vi "CD Read Engine_Parse Message.vi"(8 "Error (in)":errorcluster, 9 "Inline Status Channels Refs":T1[](array[typedef]) format="%.0x", 10 "Record []":T11[](array[typedef]) {"type" format="%04x"; "activity" format="%04x"; "error" format="%04x"; "cwd1" format="%04x"; "cwd2" format="%04x"; "swd1" format="%04x"; "swd2" format="%04x"; "data" format="%04x"}, 11 "RT Inline Data_Data Description_Channels":T2[](array[typedef]) {"Frame Drescriptors"."RT"."Status Channel Ref" format="%.0x"; "Frame Drescriptors"."RT"."Words Block Data Refs"."Data Reference" format="%.0x"; "Frame Drescriptors"."RT"."Timestamp Channel Data Reference" format="%.0x"; "Frame Drescriptors"."BC"."Status Channel Refs" format="%.0x"; "Frame Drescriptors"."BC"."Words Block Data Refs"."Data Reference" format="%.0x"; "Frame Drescriptors"."BC"."Timestamp Channel Data Reference" format="%.0x"}) -> (0 "Error (out)":errorcluster)   [LabVIEW 2017, in "Ballard MIL-1553 Engine.lvlib"]
uses:
  Ballard MIL-1553 Engine.lvlib
  <instrlib>/BTICardLib/Public/Controls/1553 Record.ctl
  Controls/RT Inline Data_Data Description_Channel.ctl
  Controls/RT Inline Frame Descriptor.ctl
  Controls/RT Inline Frame Descriptor_BC.ctl
  <vilib>/NI Veristand/Custom Device API/Data Reference.ctl
  <vilib>/NI Veristand/Custom Device API/Block Data Reference.ctl
  <vilib>/NI Veristand/Custom Device API/Custom Device Item Ref.ctl
  Controls/RT Inline Frame Descriptor_RT.ctl
  Shared/Controls and Global/RT CWD2.ctl
  Shared/Controls and Global/RT CWD1.ctl
  Shared/Controls and Global/RT messageType.ctl
  <vilib>/NI VeriStand/Custom Device Tools/Custom Device Utility Library/Custom Device Utility Library.lvlib
  <vilib>/NI VeriStand/Custom Device API/Custom Device API.lvlib
  <instrlib>/BTICardLib/BTICardLV.lvlib
  Shared/Ballard 1553 Shared.lvlib
panel:
  out "Physical Channel":u16
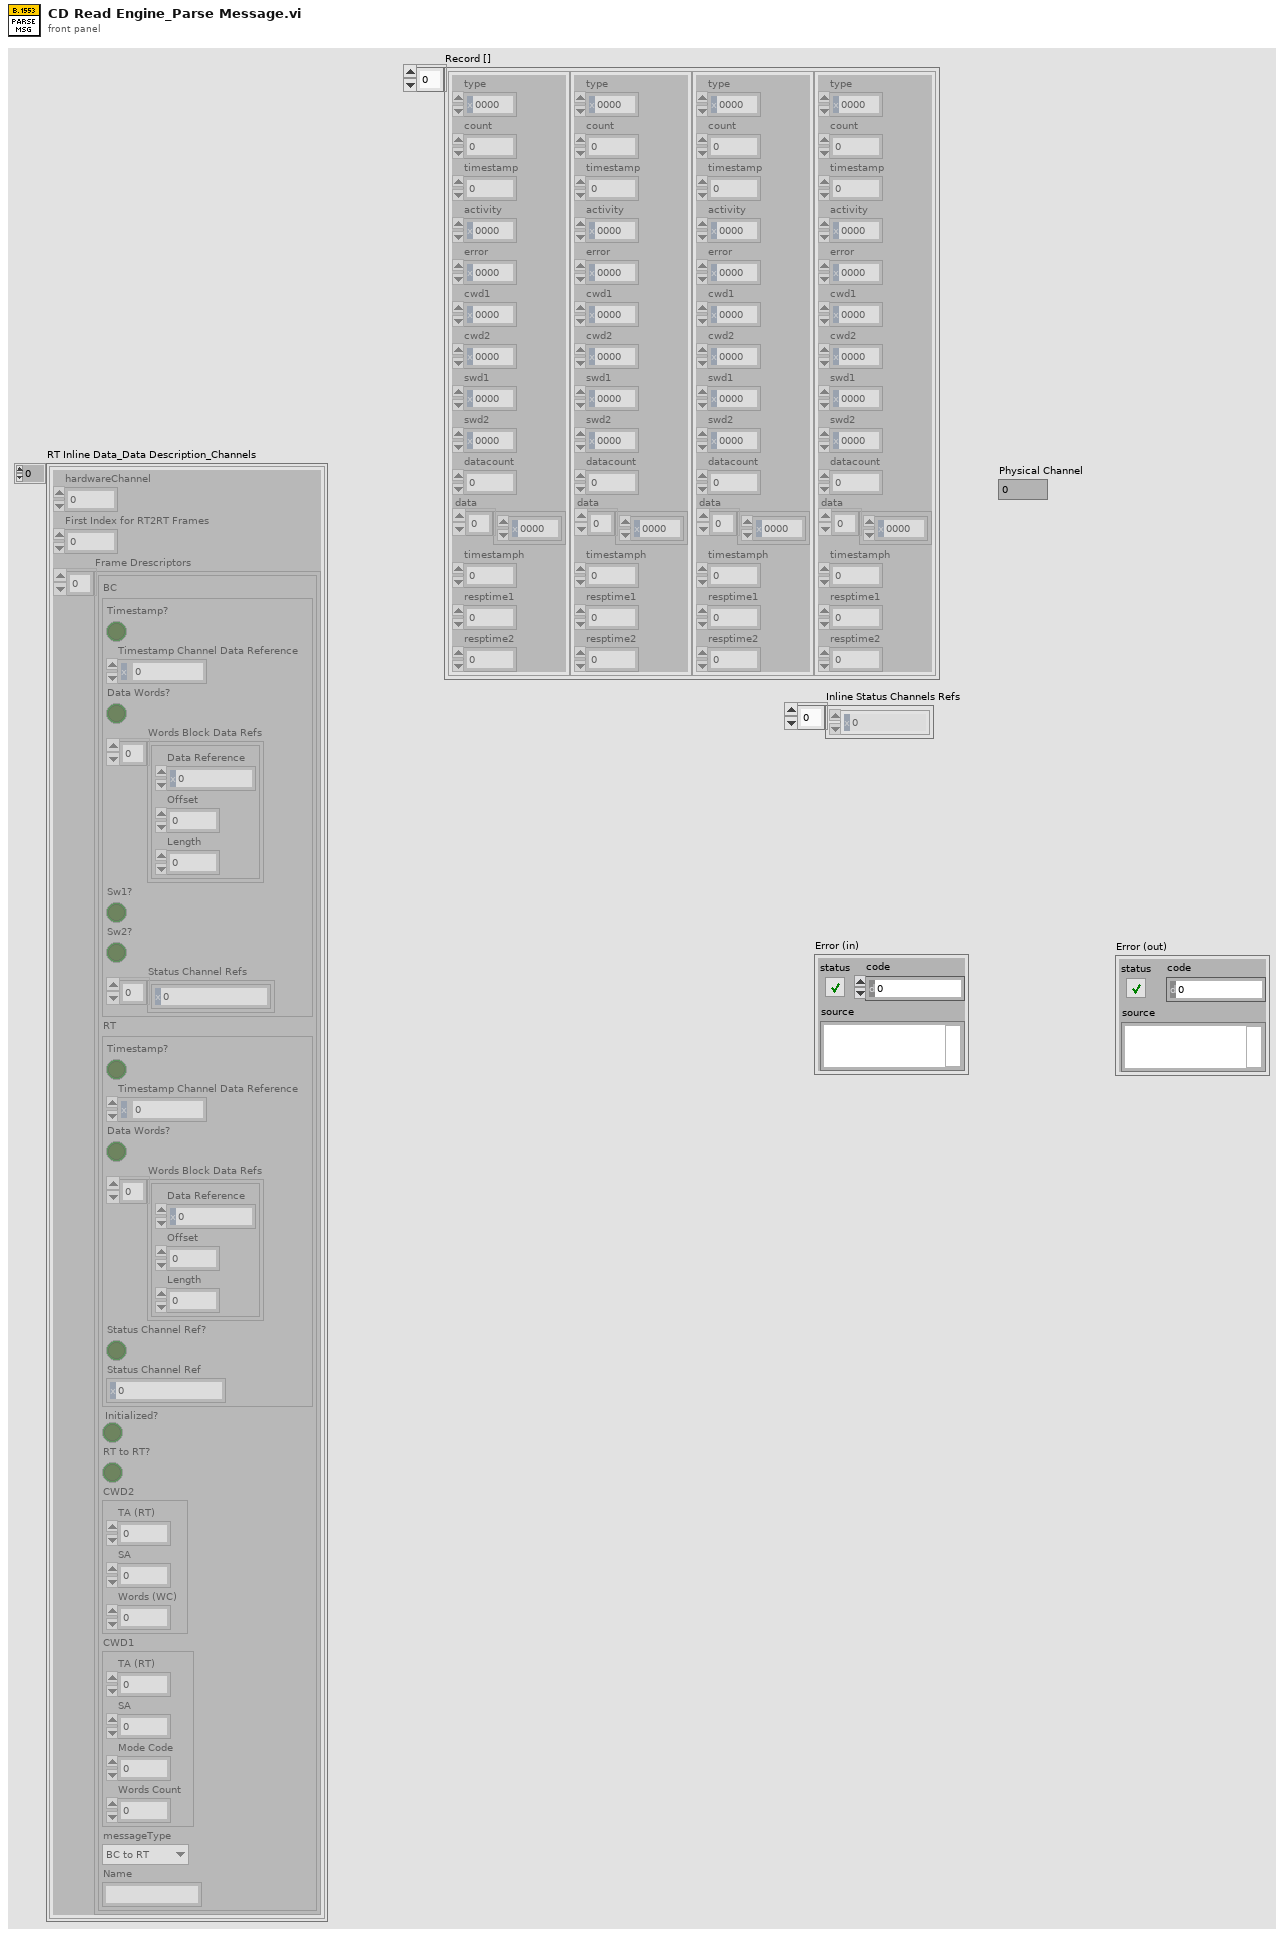
[diagram p1: front panel]
types:
  T1 = typedef "Custom Device API.lvlib/Data Reference.ctl" = i32
  T2 = typedef "Ballard MIL-1553 Engine.lvlib/RT Inline Data_Data Description_Channel.ctl" = cluster{"hardwareChannel":u16, "First Index for RT2RT Frames":i32, "Frame Drescriptors":T3[]}
  T3 = typedef "Ballard MIL-1553 Engine.lvlib/RT Inline Frame Descriptor.ctl" = cluster{"BC":T4, "RT":T7, "Initialized?":bool, "RT to RT?":bool, "CWD2":T8, "CWD1":T9, "messageType":T10, "Name":string}
  T4 = typedef "Ballard MIL-1553 Engine.lvlib/RT Inline Frame Descriptor_BC.ctl" = cluster{"Timestamp?":bool, "Timestamp Channel Data Reference":T1, "Data Words?":bool, "Words Block Data Refs":T5[], "Sw1?":bool, "Sw2?":bool, "Status Channel Refs":T6[]}
  T5 = typedef "Custom Device API.lvlib/Block Data Reference.ctl" = cluster{"Data Reference":T1, "Offset":u64, "Length":u64}
  T6 = typedef "Custom Device API.lvlib/Custom Device Item Ref.ctl" = u64
  T7 = typedef "Ballard MIL-1553 Engine.lvlib/RT Inline Frame Descriptor_RT.ctl" = cluster{"Timestamp?":bool, "Timestamp Channel Data Reference":T1, "Data Words?":bool, "Words Block Data Refs":T5[], "Status Channel Ref?":bool, "Status Channel Ref":T6}
  T8 = typedef "Ballard 1553 Shared.lvlib/RT CWD2.ctl" = cluster{"TA (RT)":i8, "SA":i8, "Words (WC)":i8}
  T9 = typedef "Ballard 1553 Shared.lvlib/RT CWD1.ctl" = cluster{"TA (RT)":i8, "SA":i8, "Mode Code":i8, "Words Count":i8}
  T10 = typedef "Ballard 1553 Shared.lvlib/RT messageType.ctl" = enum16{"BC to RT", "RT to BC", "RT to RT", "MC (Rx)", "MC (Tx)"}
  T11 = typedef "BTICardLV.lvlib/1553 Record.ctl" = cluster{"type":u16, "count":u16, "timestamp":u32, "activity":u16, "error":u16, "cwd1":u16, "cwd2":u16, "swd1":u16, "swd2":u16, "datacount":u16, "data":u16[], "timestamph":u32, "resptime1":u16, "resptime2":u16}
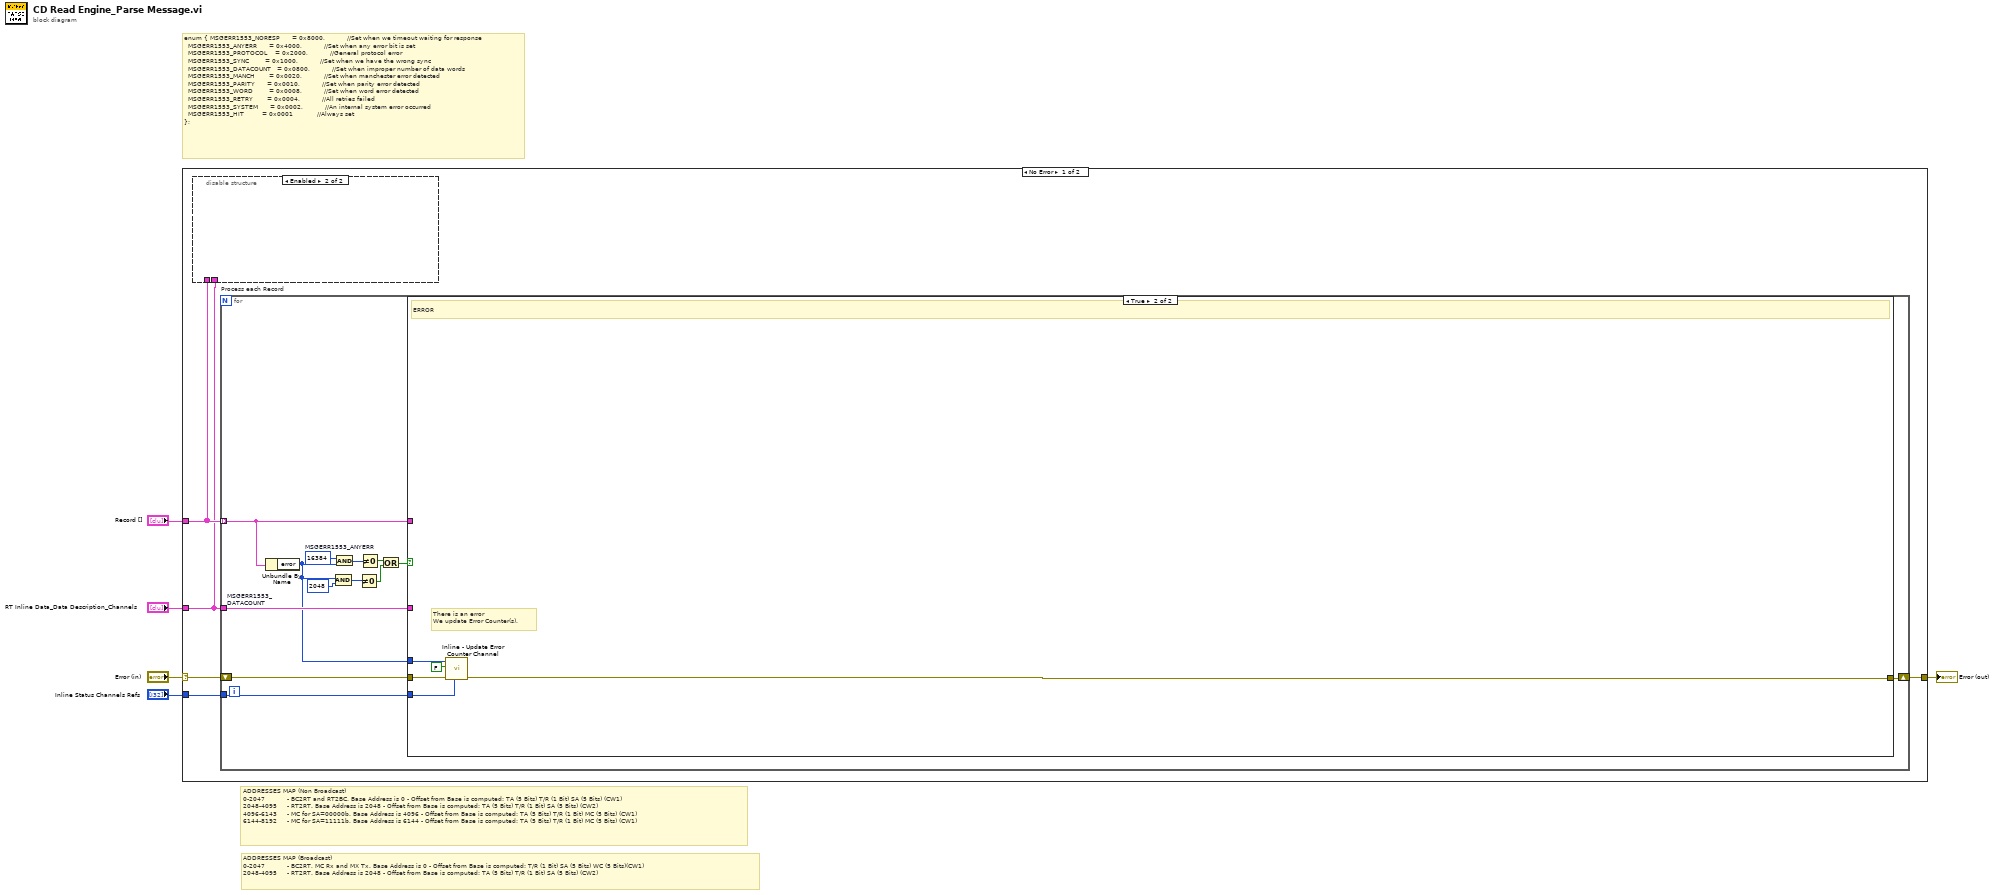
[diagram p0: block diagram]
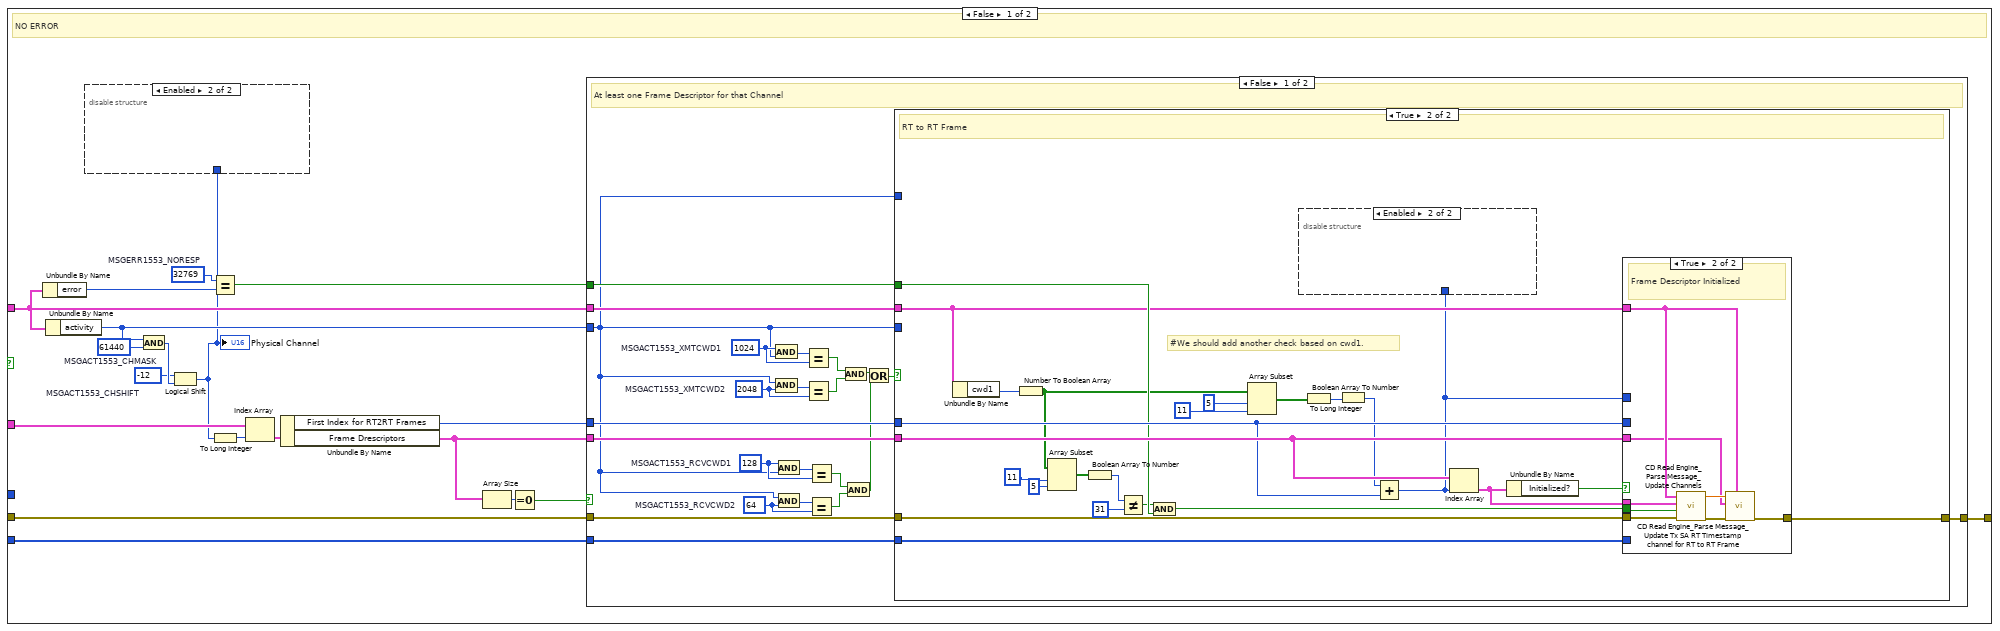
[diagram p2: hidden frame]
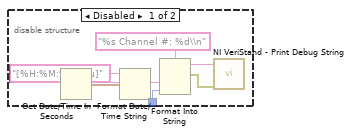
[diagram p3: hidden frame]
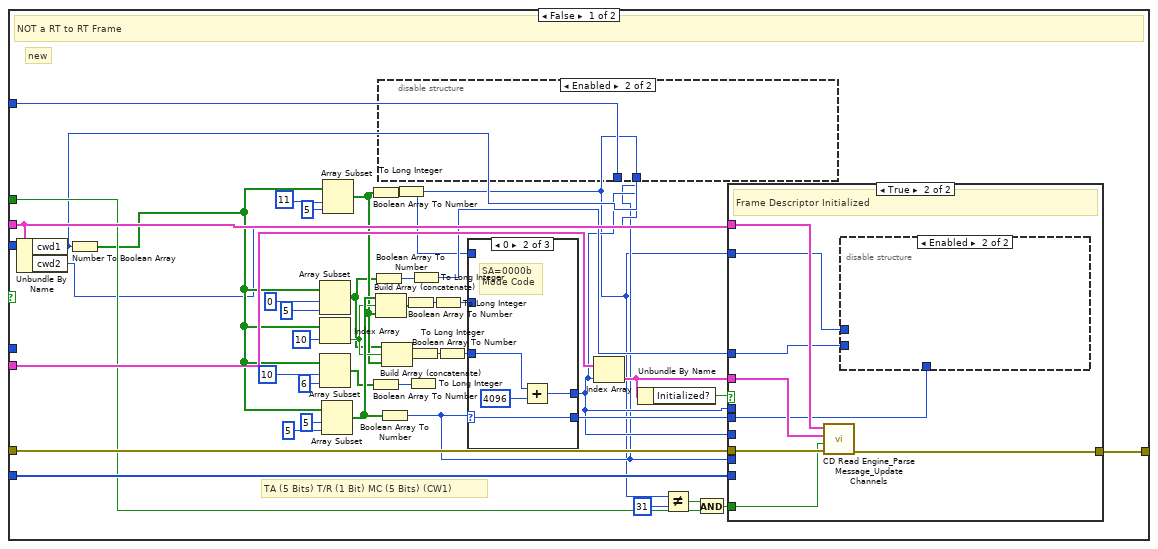
[diagram p4: hidden frame]
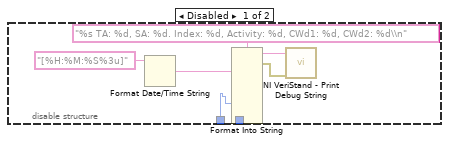
[diagram p5: hidden frame]
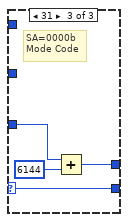
[diagram p7: hidden frame]
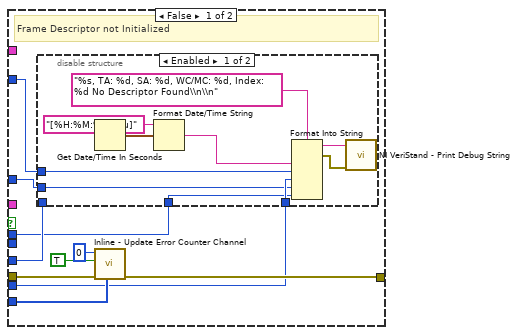
[diagram p8: hidden frame]
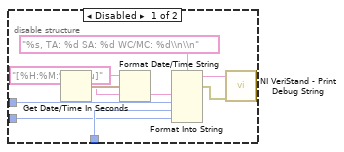
[diagram p10: hidden frame]
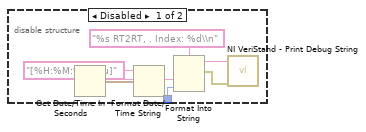
[diagram p11: hidden frame]
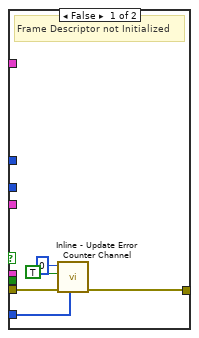
[diagram p12: hidden frame]
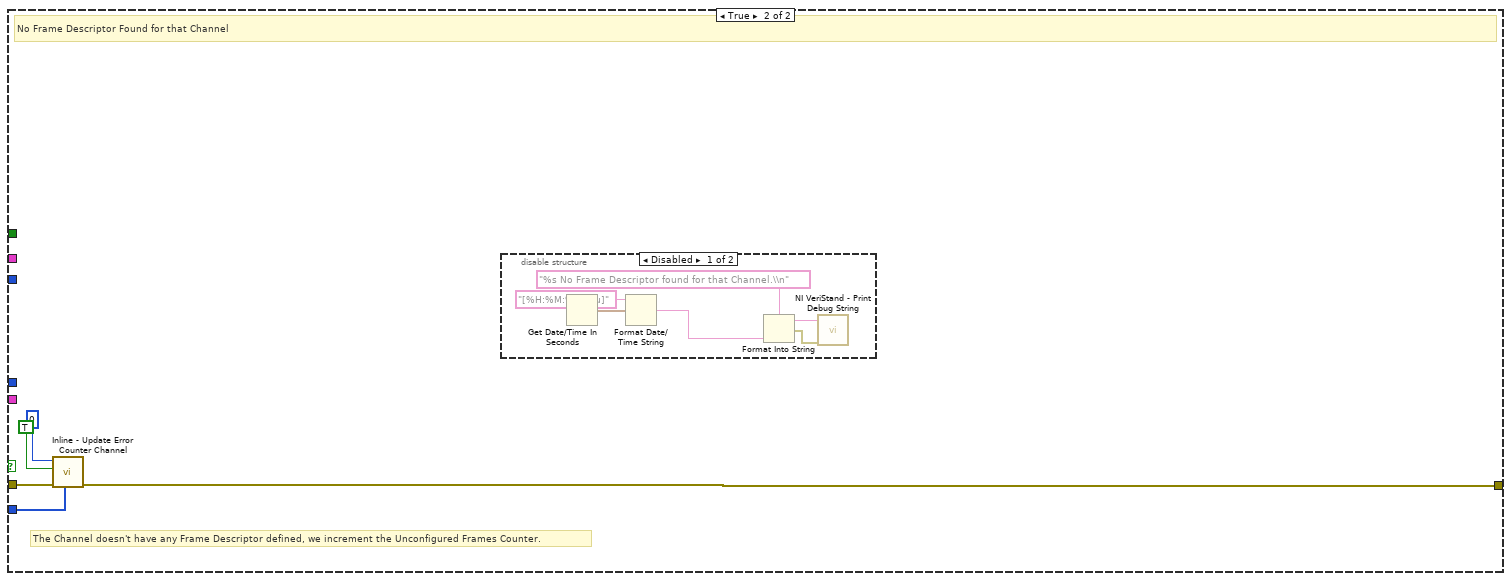
[diagram p13: hidden frame]
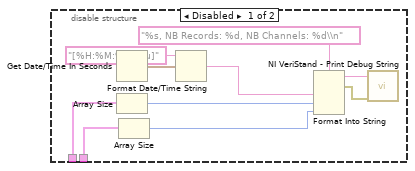
[diagram p15: hidden frame]
diagram:
  # "ADDRESSES MAP (Broadcast) \n0-2047           - BC2RT, MC Rx and MX Tx. Base Address is 0 - Offset from Base is computed: T/R (1 Bit) SA (5 Bits) WC (5 Bits)(CW1)\n2048-4095     - RT2RT. Base Address is 2048 - Offset from Base is computed: TA (5 Bits) T/R (1 Bit) SA (5 Bits) (CW2)"
  # "ADDRESSES MAP (Non Broadcast) \n0-2047           - BC2RT and RT2BC. Base Address is 0 - Offset from Base is computed: TA (5 Bits) T/R (1 Bit) SA (5 Bits) (CW1)\n2048-4095     - RT2RT. Base Address is 2048 - Offset from Base is computed: TA (5 Bits) T/R (1 Bit) SA (5 Bits) (CW2)\n4096-6143     - MC for SA=00000b. Base Address is 4096 - Offset from Base is computed: TA (5 Bits) T/R (1 Bit) MC (5 Bits) (CW1)\n6144-8192     - MC for SA=11111b. Base Address is 6144 - Offset from Base is computed: TA (5 Bits) T/R (1 Bit) MC (5 Bits) (CW1)"
  # "enum {\tMSGERR1553_NORESP      = 0x8000,           //Set when we timeout waiting for response\n\t\tMSGERR1553_ANYERR      = 0x4000,           //Set when any error bit is set\n\t\tMSGERR1553_PROTOCOL    = 0x2000,           //General protocol error\n\t\tMSGERR1553_SYNC        = 0x1000,           //Set when we have the wrong sync\n\t\tMSGERR1553_DATACOUNT   = 0x0800,           //Set when improper number of data words\n\t\tMSGERR1553_MANCH       = 0x0020,           //Set when manchester error detected\n\t\tMSGERR1553_PARITY      = 0x0010,           //Set when parity error detected\n\t\tMSGERR1553_WORD        = 0x0008,           //Set when word error detected\n\t\tMSGERR1553_RETRY       = 0x0004,           //All retries failed\n\t\tMSGERR1553_SYSTEM      = 0x0002,           //An internal system error occurred\n\t\tMSGERR1553_HIT         = 0x0001            //Always set\n};"
  n1 = case shown="No Error" "Error (in)" {
    selector: "Error (in)" -> [w9 w244]
    tunnel: "Record []" -> [w8 _]
    tunnel: [w10 w244] -> w4
    tunnel: "RT Inline Data_Data Description_Channels" -> [w6 _]
    tunnel: "Inline Status Channels Refs" -> [w7 _]
    frame No Error {
      n2 = disable-structure shown="Enabled" {
        disable-tunnel: w8 -> [w243 _]
        disable-tunnel: w6 -> [w235 _]
        frame Disabled {
          n3 = Get Date/Time In Seconds() -> (seconds since 1Jan1904=w242:timestamp)
          n4 = Array Size(array=w243) -> (size(s)=w240:i32)
          n5 = Array Size(array=w235) -> (size(s)=w234:i32)
          n6 = Format Date/Time String(time format string (%c)="[%H:%M:%S%3u]", seconds (now)=w242) -> (date/time string=w241:string)  [unwired: 1 in]
          n7 = Format Into String(format string="%s, NB Records: %d, NB Channels: %d\\n", w241, w240, w234) -> (resulting string=w236:string, error out=w237:errorcluster)  [unwired: 2 in]
          n8 = call <vilib>:"NI VeriStand - Print Debug String.vi"("error in (no error)"=w237, "Message"=w236) -> ()  [unwired: 9 in, 1 out]
        }
        frame Enabled {
        }
      }
      n9 = for "Process each Record" {
        tunnel: w8 -> [w23] mode=indexing
        shift-right: [w22] -> w10
        shift-left: w9 -> [w21]
        tunnel: w7 -> [w20]
        tunnel: w6 -> [w19]
        w11 = u16 2048  # MSGERR1553_DATACOUNT
        w18 = u16 16384  # MSGERR1553_ANYERR
        n10 = Unbundle By Name(w23) -> ("error"=w14:u16)
        n11 = And(x=w14, y=w11) -> (x .and. y?=w13:u16)
        n12 = And(x=w18, y=w14) -> (x .and. y?=w17:u16)
        n13 = Not Equal To 0?(x=w13) -> (x != 0?=w12:bool)
        n14 = Not Equal To 0?(x=w17) -> (x != 0?=w16:bool)
        n15 = Or(x=w16, y=w12) -> (x .or. y?=w15:bool)
        n16 = case "Channel Found?" shown="True" w15 {
          tunnel: w21 -> [w41 w232]
          tunnel: [w42 w230] -> w22
          tunnel: w23 -> [w29 _]
          tunnel: w20 -> [w32 w231]
          tunnel: w19 -> [w39 _]
          tunnel: w14 -> [_ w233]
          frame False {
            w27 = u16 32769  # MSGERR1553_NORESP
            w30 = i16 -12  # MSGACT1553_CHSHIFT
            w40 = u16 61440  # MSGACT1553_CHMASK
            # "NO ERROR"
            n17 = Unbundle By Name(w29) -> ("error"=w28:u16)
            n18 = Unbundle By Name(w29) -> ("activity"=w34:u16)
            n19 = And(x=w34, y=w40) -> (x .and. y?=w31:u16)
            n20 = Logical Shift(y=w30, x=w31) -> (x << y=w25:u16)
            "Physical Channel" <- w25
            n21 = disable-structure shown="Enabled" {
              disable-tunnel: w25 -> [w43 _]
              frame Disabled {
                n22 = Get Date/Time In Seconds() -> (seconds since 1Jan1904=w49:timestamp)
                n23 = Format Date/Time String(time format string (%c)="[%H:%M:%S%3u]", seconds (now)=w49) -> (date/time string=w48:string)  [unwired: 1 in]
                n24 = Format Into String(format string="%s Channel #: %d\\n", w48, w43) -> (resulting string=w44:string, error out=w45:errorcluster)  [unwired: 2 in]
                n25 = call <vilib>:"NI VeriStand - Print Debug String.vi"("error in (no error)"=w45, "Message"=w44) -> ()  [unwired: 9 in, 1 out]
              }
              frame Enabled {
              }
            }
            n26 = Equal?(x=w27, y=w28) -> (x = y?=w26:bool)
            n27 = To Long Integer(number=w25) -> (32bit integer=w38:i32)
            n28 = Index Array(array=w39, index=w38) -> (element=w36:T2)
            n29 = Unbundle By Name(w36) -> ("First Index for RT2RT Frames"=w33:i32, "Frame Drescriptors"=w35:T3[])
            n30 = Array Size(array=w35) -> (size(s)=w37:i32)
            n31 = Equal To 0?(x=w37) -> (x = 0?=w24:bool)
            n32 = case shown="False" w24 {
              tunnel: [w72 w218] -> w42
              tunnel: w29 -> [w71 _]
              tunnel: w41 -> [w70 w221]
              tunnel: w35 -> [w63 _]
              tunnel: w34 -> [w50 _]
              tunnel: w33 -> [w64 _]
              tunnel: w32 -> [w62 w220]
              tunnel: w26 -> [w60 _]
              frame False {
                w59 = u16 128  # MSGACT1553_RCVCWD1
                w58 = u16 64  # MSGACT1553_RCVCWD2
                w61 = u16 1024  # MSGACT1553_XMTCWD1
                w65 = u16 2048  # MSGACT1553_XMTCWD2
                # "At least one Frame Descriptor for that Channel"
                n33 = And(x=w61, y=w50) -> (x .and. y?=w68:u16)
                n34 = And(x=w50, y=w65) -> (x .and. y?=w66:u16)
                n35 = And(x=w59, y=w50) -> (x .and. y?=w55:u16)
                n36 = And(x=w50, y=w58) -> (x .and. y?=w57:u16)
                n37 = Equal?(x=w68, y=w61) -> (x = y?=w69:bool)
                n38 = Equal?(x=w66, y=w65) -> (x = y?=w67:bool)
                n39 = Equal?(x=w55, y=w59) -> (x = y?=w54:bool)
                n40 = Equal?(x=w57, y=w58) -> (x = y?=w56:bool)
                n41 = And(x=w69, y=w67) -> (x .and. y?=w52:bool)
                n42 = And(x=w54, y=w56) -> (x .and. y?=w51:bool)
                n43 = Or(x=w52, y=w51) -> (x .or. y?=w53:bool)
                n44 = case shown="True" w53 {
                  tunnel: w71 -> [w113 w191]
                  tunnel: w70 -> [w114 w196]
                  tunnel: [w115 w197] -> w72
                  tunnel: w64 -> [_ w193]
                  tunnel: w63 -> [w112 w195]
                  tunnel: w62 -> [w111 w194]
                  tunnel: w60 -> [w110 w192]
                  tunnel: w50 -> [_ _]
                  tunnel: w50 -> [w109 _]
                  frame False {
                    # "TA (5 Bits) T/R (1 Bit) MC (5 Bits) (CW1)"
                    # "new"
                    # "NOT a RT to RT Frame"
                    n45 = Unbundle By Name(w113) -> ("cwd1"=w107:u16, "cwd2"=w106:u16)
                    n46 = Number To Boolean Array(number=w107) -> (Boolean array=w108:bool[])
                    n47 = Array Subset(array=w108, index=0, length=5) -> (w81:bool[])
                    n48 = Index Array(array=w108, index=10) -> (element=w84:bool)
                    n49 = Array Subset(array=w108, index=10, length=6) -> (w79:bool[])
                    n50 = Array Subset(array=w108, index=5, length=5) -> (w85:bool[])
                    n51 = Array Subset(array=w108, index=11, length=5) -> (w83:bool[])
                    n52 = Boolean Array To Number(Boolean array=w83) -> (number=w90:u32)
                    n53 = Boolean Array To Number(Boolean array=w79) -> (number=w80:u32)
                    n54 = Boolean Array To Number(Boolean array=w81) -> (number=w94:u32)
                    n55 = Build Array (concatenate)(w85, w84, w83) -> (w99:bool[])
                    n56 = Boolean Array To Number(Boolean array=w85) -> (number=w77:u16)
                    n57 = Build Array (concatenate)(w81, w84, w83) -> (w82:bool[])
                    n58 = To Long Integer(number=w90) -> (32bit integer=w75:i32)
                    n59 = Boolean Array To Number(Boolean array=w99) -> (number=w96:u16)
                    n60 = To Long Integer(number=w80) -> ()  [unwired: 1 out]
                    n61 = Boolean Array To Number(Boolean array=w82) -> (number=w87:u16)
                    n62 = To Long Integer(number=w94) -> (32bit integer=w93:i32)
                    n63 = To Long Integer(number=w96) -> (32bit integer=w89:i32)
                    n64 = To Long Integer(number=w87) -> (32bit integer=w86:i32)
                    n65 = case shown="0" w77 {
                      selector: w77 -> [w128 w130 w134]
                      tunnel: w75 -> [_ _ _]
                      tunnel: [w127 w132 w136] -> w78
                      tunnel: w89 -> [w127 _ _]
                      tunnel: [w128 w130 w134] -> w95
                      tunnel: w86 -> [_ w129 w133]
                      frame 1, Default {
                      }
                      frame 0 {
                        # "SA=0000b\nMode Code"
                        n66 = Add(x=w129, y=4096) -> (x+y=w132:i32)
                      }
                      frame 31 {
                        # "SA=0000b\nMode Code"
                        n67 = Add(x=w133, y=6144) -> (x+y=w136:i32)
                      }
                    }
                    n68 = disable-structure shown="Enabled" {
                      disable-tunnel: w75 -> [w122 _]
                      disable-tunnel: w78 -> [w121 _]
                      disable-tunnel: w77 -> [w119 _]
                      disable-tunnel: w109 -> [w118 _]
                      disable-tunnel: w107 -> [w117 _]
                      disable-tunnel: w106 -> [w116 _]
                      frame Disabled {
                        n69 = Format Date/Time String(time format string (%c)="[%H:%M:%S%3u]") -> (date/time string=w126:string)  [unwired: 2 in]
                        n70 = Format Into String(format string="%s TA: %d, SA: %d. Index: %d, Activity: %d, CWd1: %d, CWd2: %d\\n", w126, w122, w119, w121, w118, w117, w116) -> (resulting string=w123:string, error out=w124:errorcluster)  [unwired: 2 in]
                        n71 = call <vilib>:"NI VeriStand - Print Debug String.vi"("error in (no error)"=w124, "Message"=w123) -> ()  [unwired: 9 in, 1 out]
                      }
                      frame Enabled {
                      }
                    }
                    n72 = Index Array(array=w112, index=w78) -> (element=w105:T3)
                    n73 = Unbundle By Name(w105) -> ("Initialized?"=w104:bool)
                    n74 = Not Equal?(x=w75, y=31) -> (x != y?=w76:bool)
                    n75 = And(x=w76, y=w110) -> (x .and. y?=w73:bool)
                    n76 = case shown="True" w104 {
                      tunnel: [w143 w164] -> w115
                      tunnel: w114 -> [w144 w163]
                      tunnel: w113 -> [_ w162]
                      tunnel: w105 -> [_ w161]
                      tunnel: w111 -> [w142 _]
                      tunnel: w75 -> [w141 w160]
                      tunnel: w95 -> [_ w159]
                      tunnel: w93 -> [w138 w158]
                      tunnel: w78 -> [w140 _]
                      tunnel: w77 -> [w139 _]
                      tunnel: w78 -> [w137 _]
                      tunnel: w73 -> [_ w157]
                      frame False {
                        # "Frame Descriptor not Initialized"
                        n77 = disable-structure shown="Enabled" {
                          disable-tunnel: w141 -> [w150 _]
                          disable-tunnel: w140 -> [_ _]
                          disable-tunnel: w139 -> [w149 _]
                          disable-tunnel: w138 -> [w148 _]
                          disable-tunnel: w137 -> [w147 _]
                          frame Enabled {
                            n78 = Get Date/Time In Seconds() -> (seconds since 1Jan1904=w156:timestamp)
                            n79 = Format Date/Time String(time format string (%c)="[%H:%M:%S%3u]", seconds (now)=w156) -> (date/time string=w155:string)  [unwired: 1 in]
                            n80 = Format Into String(format string="%s, TA: %d, SA: %d, WC/MC: %d, Index: %d No Descriptor Found\\n\\n", w155, w150, w149, w148, w147) -> (resulting string=w151:string, error out=w152:errorcluster)  [unwired: 2 in]
                            n81 = call <vilib>:"NI VeriStand - Print Debug String.vi"("error in (no error)"=w152, "Message"=w151) -> ()  [unwired: 9 in, 1 out]
                          }
                          frame Disabled {
                          }
                        }
                        n82 = call "Inline - Update Error Counter Channel.vi"("Inline Status Channels Refs"=w142, "error in (no error)"=w144, "Increment Unconfigured Frames Counter?"=TRUE, "error"=u16 0) -> ("error IO"=w143:errorcluster)  [unwired: 6 in, 1 out]
                      }
                      frame True {
                        # "Frame Descriptor Initialized"
                        n83 = call "CD Read Engine_Parse Message_Update Channels.vi"("error in (no error)"=w163, "NORESP"=w157, "Frame Descriptor"=w161, "record in"=w162) -> ("error out"=w164:errorcluster)  [unwired: 6 in, 1 out]
                        n84 = disable-structure shown="Enabled" {
                          disable-tunnel: w160 -> [w167 _]
                          disable-tunnel: w159 -> [w166 _]
                          disable-tunnel: w158 -> [w165 _]
                          frame Disabled {
                            n85 = Get Date/Time In Seconds() -> (seconds since 1Jan1904=w173:timestamp)
                            n86 = Format Date/Time String(time format string (%c)="[%H:%M:%S%3u]", seconds (now)=w173) -> (date/time string=w172:string)  [unwired: 1 in]
                            n87 = Format Into String(format string="%s, TA: %d SA: %d WC/MC: %d\\n\\n", w172, w167, w166, w165) -> (resulting string=w168:string, error out=w169:errorcluster)  [unwired: 2 in]
                            n88 = call <vilib>:"NI VeriStand - Print Debug String.vi"("error in (no error)"=w169, "Message"=w168) -> ()  [unwired: 9 in, 1 out]
                          }
                          frame Enabled {
                          }
                        }
                      }
                    }
                  }
                  frame True {
                    # "#We should add another check based on cwd1."
                    # "RT to RT Frame"
                    n89 = Unbundle By Name(w191) -> ("cwd1"=w188:u16)
                    n90 = Number To Boolean Array(number=w188) -> (Boolean array=w175:bool[])
                    n91 = Array Subset(array=w175, index=11, length=5) -> (w176:bool[])
                    n92 = Boolean Array To Number(Boolean array=w176) -> (number=w174:u32)
                    n93 = Not Equal?(x=w174, y=u32 31) -> (x != y?=w181:bool)
                    n94 = And(x=w181, y=w192) -> (x .and. y?=w179:bool)
                    n95 = Array Subset(array=w175, index=5, length=11) -> (w187:bool[])
                    n96 = Boolean Array To Number(Boolean array=w187) -> (number=w186:u32)
                    n97 = To Long Integer(number=w186) -> (32bit integer=w185:i32)
                    n98 = Add(x=w185, y=w193) -> (x+y=w183:i32)
                    n99 = disable-structure shown="Enabled" {
                      disable-tunnel: w183 -> [w198 _]
                      frame Disabled {
                        n100 = Get Date/Time In Seconds() -> (seconds since 1Jan1904=w204:timestamp)
                        n101 = Format Date/Time String(time format string (%c)="[%H:%M:%S%3u]", seconds (now)=w204) -> (date/time string=w203:string)  [unwired: 1 in]
                        n102 = Format Into String(format string="%s RT2RT, . Index: %d\\n", w203, w198) -> (resulting string=w199:string, error out=w200:errorcluster)  [unwired: 2 in]
                        n103 = call <vilib>:"NI VeriStand - Print Debug String.vi"("error in (no error)"=w200, "Message"=w199) -> ()  [unwired: 9 in, 1 out]
                      }
                      frame Enabled {
                      }
                    }
                    n104 = Index Array(array=w195, index=w183) -> (element=w184:T3)
                    n105 = Unbundle By Name(w184) -> ("Initialized?"=w182:bool)
                    n106 = case shown="True" w182 {
                      tunnel: [w206 w212] -> w197
                      tunnel: w196 -> [w207 w217]
                      tunnel: w191 -> [_ w214]
                      tunnel: w184 -> [_ w216]
                      tunnel: w194 -> [w205 _]
                      tunnel: w183 -> [_ _]
                      tunnel: w179 -> [_ w215]
                      tunnel: w195 -> [_ w210]
                      tunnel: w193 -> [_ _]
                      frame False {
                        # "Frame Descriptor not Initialized"
                        n107 = call "Inline - Update Error Counter Channel.vi"("Inline Status Channels Refs"=w205, "error in (no error)"=w207, "Increment Unconfigured Frames Counter?"=TRUE, "error"=u16 0) -> ("error IO"=w206:errorcluster)  [unwired: 6 in, 1 out]
                      }
                      frame True {
                        # "Frame Descriptor Initialized"
                        n108 = call "CD Read Engine_Parse Message_Update Channels.vi"("error in (no error)"=w217, "NORESP"=w215, "Frame Descriptor"=w216, "record in"=w214) -> ("error out"=w213:errorcluster, "Timestamp (s)"=w211:dbl)  [unwired: 6 in]
                        n109 = call "CD Read Engine_Parse Message_Update Tx SA RT Timestamp channel for RT to RT Frame.vi"("record in"=w214, "error in (no error)"=w213, "Frame Drescriptors"=w210, "Timestamp (s)"=w211) -> ("error out"=w212:errorcluster)  [unwired: 7 in]
                      }
                    }
                  }
                }
              }
              frame True {
                # "The Channel doesn't have any Frame Descriptor defined, we increment the Unconfigured Frames Counter."
                # "No Frame Descriptor Found for that Channel"
                n110 = call "Inline - Update Error Counter Channel.vi"("Inline Status Channels Refs"=w220, "error in (no error)"=w221, "Increment Unconfigured Frames Counter?"=TRUE, "error"=u16 0) -> ("error IO"=w218:errorcluster)  [unwired: 6 in, 1 out]
                n111 = disable-structure shown="Disabled" {
                  frame Disabled {
                    n112 = Get Date/Time In Seconds() -> (seconds since 1Jan1904=w228:timestamp)
                    n113 = Format Date/Time String(time format string (%c)="[%H:%M:%S%3u]", seconds (now)=w228) -> (date/time string=w227:string)  [unwired: 1 in]
                    n114 = Format Into String(format string="%s No Frame Descriptor found for that Channel.\\n", w227) -> (resulting string=w223:string, error out=w224:errorcluster)  [unwired: 2 in]
                    n115 = call <vilib>:"NI VeriStand - Print Debug String.vi"("error in (no error)"=w224, "Message"=w223) -> ()  [unwired: 9 in, 1 out]
                  }
                  frame Enabled {
                  }
                }
              }
            }
          }
          frame True {
            # "There is an error\nWe update Error Counter(s)."
            # "ERROR"
            n116 = call "Inline - Update Error Counter Channel.vi"("Inline Status Channels Refs"=w231, "error in (no error)"=w232, "Increment Unconfigured Frames Counter?"=FALSE, "error"=w233) -> ("error IO"=w230:errorcluster)  [unwired: 6 in, 1 out]
          }
        }
      }
    }
    frame Error {
    }
  }
  "Error (out)" <- w4
